vi "LabVIEW Basics #5 - Radar Sweep.vi"() -> ()   [LabVIEW 2019]
uses:
  <vilib>/picture/picture.llb/imagedata.ctl
  <vilib>/MakerHub/LINX/Public/Utilities/Open Serial.vi
  <vilib>/MakerHub/LINX/Public/Sensors/Motion/Servo/Servo Open One Channel.vi
  <vilib>/MakerHub/LINX/Public/Sensors/Motion/Servo/Servo Set Pulse Width One Channel.vi
  <vilib>/MakerHub/LINX/Public/Sensors/Motion/Servo/Servo Close One Channel.vi
  <vilib>/MakerHub/LINX/LMH-LINX.lvlib
  <vilib>/MakerHub/LINX/Public/Sensors/Motion/Servo/Servo.lvlib
  <vilib>/MakerHub/LINX/Public/Sensors/Distance/Ultrasonic/Ultrasonic.lvlib
  <vilib>/ptbypt/NI_PtbyPt.lvlib
panel:
  out "ping":bool
  out "Degrees":dbl format="%#_3f"
  out "Distance":dbl caption="CM" format="%#_2g"
  out "2D Picture":picture
  out "Device Name":string
  in  "Stop":bool
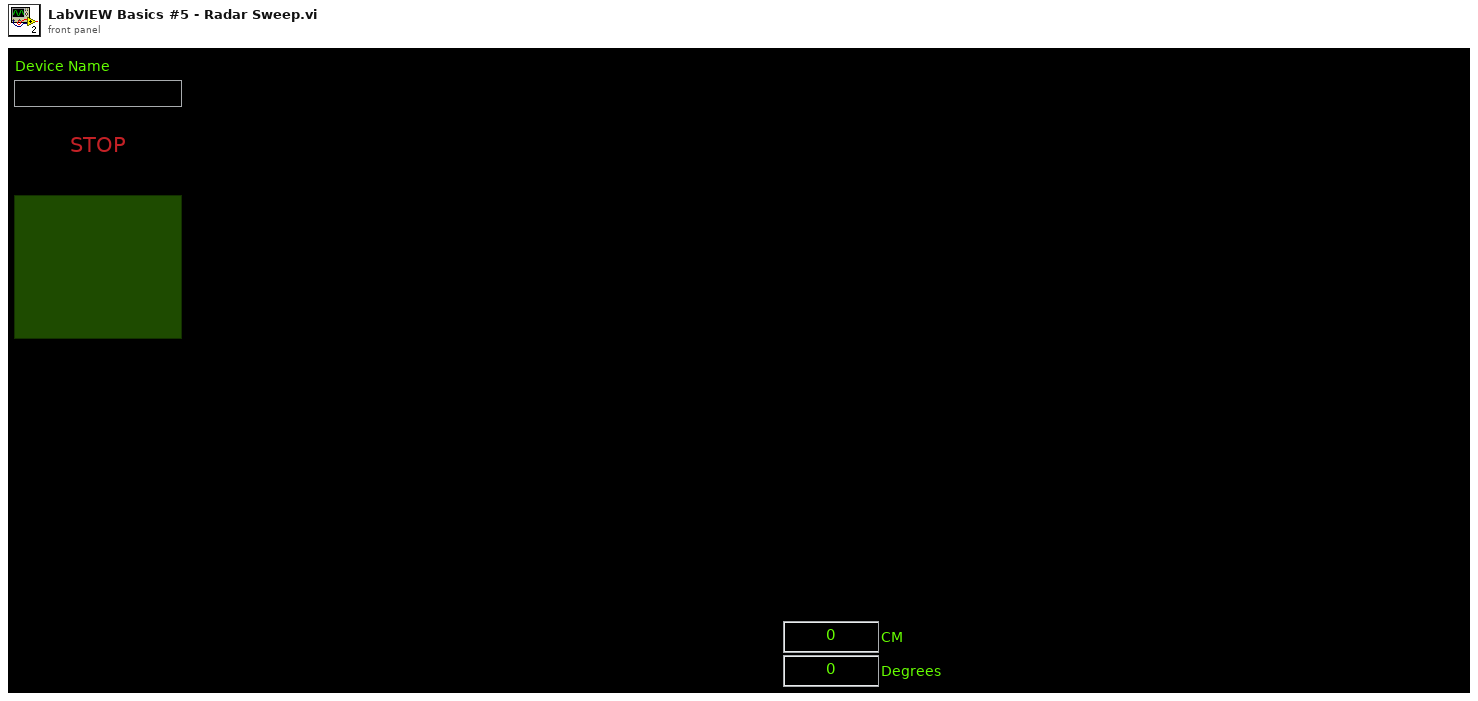
[diagram p1: front panel]
types:
  T1 = typedef "imagedata.ctl" = cluster{"image type":i32, "image depth":i32, "image":u8[], "mask":u8[], "colors":u32[], "Rectangle":cluster{"left":i16, "top":i16, "right":i16, "bottom":i16}}
  T2 = typedef "LMH-LINX.lvlib/LINX Ref.ctl" = cluster{"IO":T3, "Interface":T4, "LINX Device Config":T5}
  T3 = typedef "LMH-LINX.lvlib/Platform.ctl" = enum16{"Remote", "Local"}
  T4 = typedef "LMH-LINX.lvlib/Interface.ctl" = enum16{"Serial", "TCP"}
  T5 = typedef "LMH-LINX.lvlib/Device.lvlib/LINX Device Config.ctl" = cluster{"Interface":T4, "COM Port":refnum<visa-resource-name>, "TCP Configuration":T6, "Device Family":u8, "Device ID":u8, "Device Name":string, "TCP Ref":refnum<k5>, "Channels":T7}
  T6 = typedef "LMH-LINX.lvlib/Device.lvlib/TCP Config.ctl" = cluster{"IP Address":string, "Port":u16}
  T7 = typedef "LMH-LINX.lvlib/Channels.ctl" = cluster{"DI":u8[], "DO":u8[], "AI":u8[], "AO":u8[], "PWM":u8[], "QE":u8[], "UART":u8[], "I2C 2":u8[], "SPI":u8[], "CAN":u8[], "Servo":u8[], "AI Ref (V)":dbl, "AI Resolution (Bits)":u8, "AO Ref (V)":dbl, "AO Resolution (Bits)":u8}
  T8 = cluster{"maximum":dbl, "minimum":dbl, "clip to min":bool, "log?(F)":bool, "grid color":u32, "plot color":u32, "format and precision":cluster{"format":enum8{"Decimal", "Scientific", "Engineering", "Binary", "Octal", "Hex"}, "precision":u8}, "visible section":u16}
  T9 = typedef "LVBoundsTypeDef.ctl" = cluster{"Width":u32, "Height":u32}
  T10 = cluster{"pixel center":cluster{"x":i16, "y":i16}, "scale factors":cluster{"a":dbl, "b":dbl, "log?":bool}, "grid color":u32, "start angle":dbl, "end angle":dbl, "tick length":i16, "pixel radius":i32}
  T11 = cluster{"Distance (cm)":dbl, "Angle (Deg)":dbl}[]
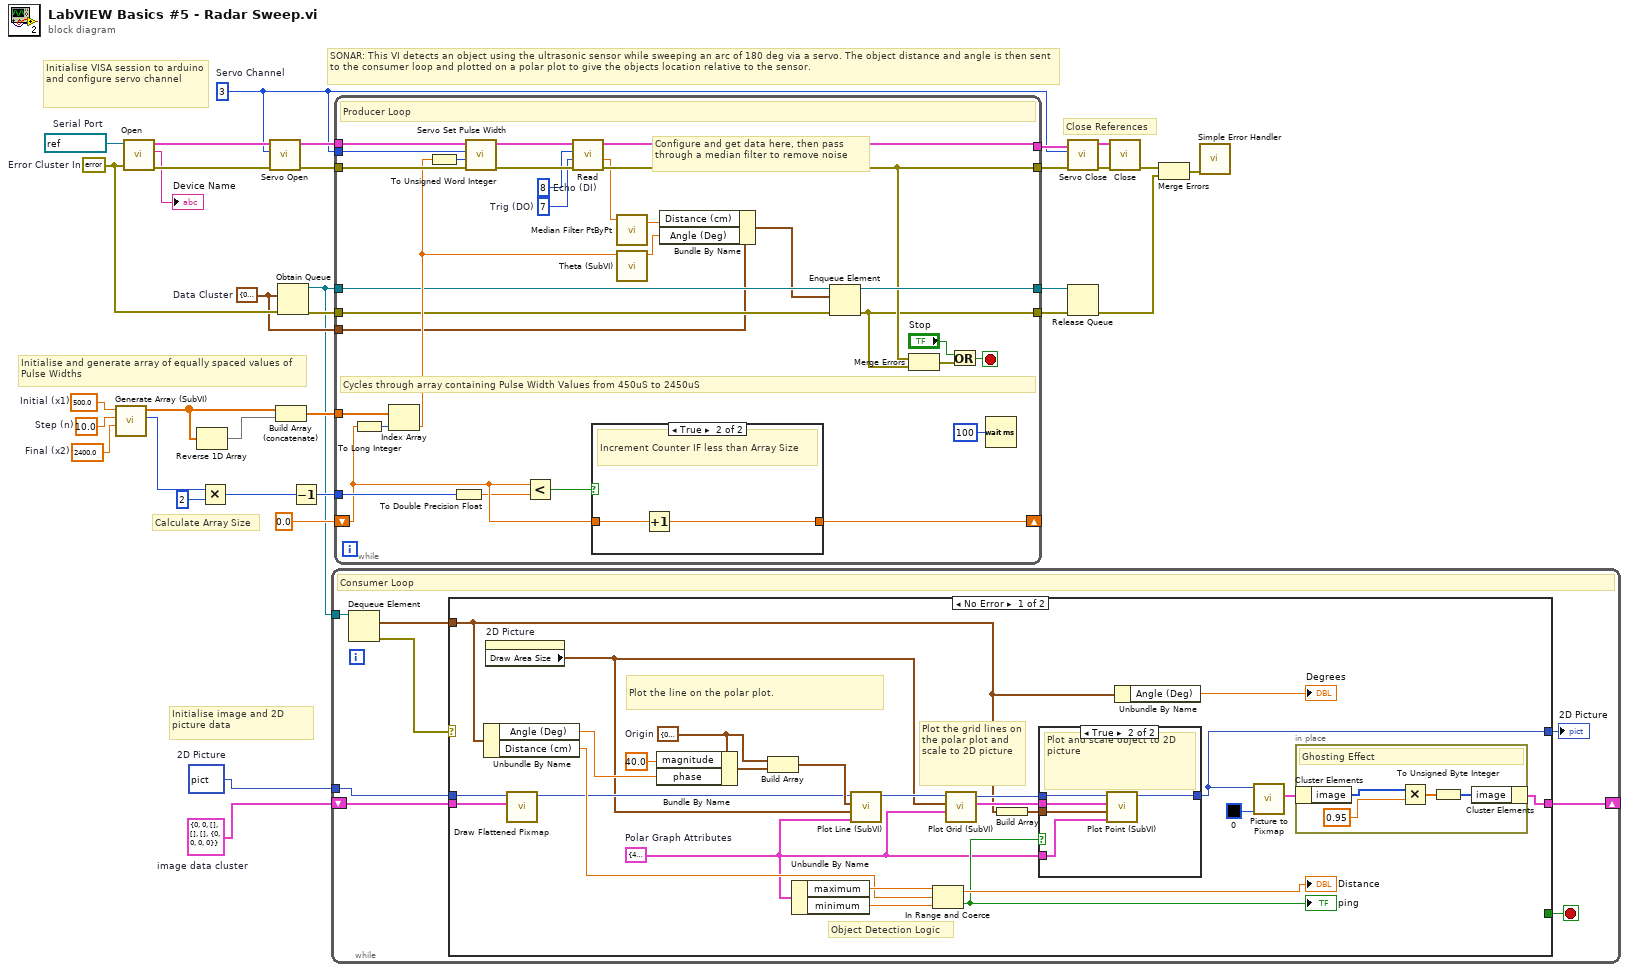
[diagram p0: block diagram]
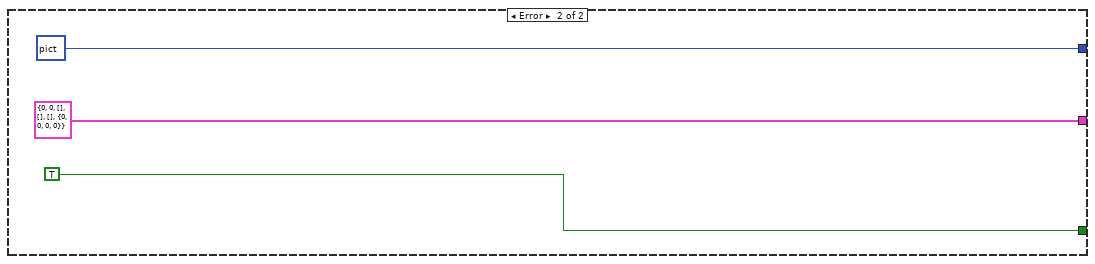
[diagram p3: hidden frame]
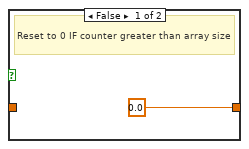
[diagram p4: hidden frame]
diagram:
  w1 = T1 {"image type"=0, "image depth"=0, "image"=[], "mask"=[], "colors"=[], "Rectangle"={"left"=0, "top"=0, "right"=0, "bottom"=0}}  # image data cluster
  w2 = picture data[5B]  # 2D Picture
  w7 = cluster{"Distance (cm)":dbl, "Angle (Deg)":dbl} {"Distance (cm)"=0.0, "Angle (Deg)"=0.0}  # Data Cluster
  w21 = 2400.0  # Final (x2)
  w20 = 10.0  # Step (n)
  w19 = 500.0  # Initial (x1)
  w24 = u8 3  # Servo Channel
  w10 = errorcluster {"status"=FALSE, "code"=0, "source"=""}  # Error Cluster In
  w33 = refnum<visa-resource-name> "COM6"  # Serial Port
  # "Initialise image and 2D picture data"
  # "Close References"
  # "Calculate Array Size"
  # "Initialise and generate array of equally spaced values of Pulse Widths"
  # "Initialise VISA session to arduino and configure servo channel"
  # "SONAR: This VI detects an object using the ultrasonic sensor while sweeping an arc of 180 deg via a servo. The object distance and angle is then sent to the consumer loop and plotted on a polar plot to give the objects location relative to the sensor."
  n1 = call "Generate Array (SubVI).vi"("Final"=w21, "Step"=w20, "Initial"=w19) -> ("Array size"=w14:i32, "Array out"=w17:dbl[])  [unwired: 6 in, 1 out]
  n2 = call-poly <vilib>:"Open.vi"("Error In"=w10, "Serial Port"=w33) -> ("Error Out"=w29:errorcluster, "Device Name"=→"Device Name":string, "LINX Resource"=w30:T2)  [unwired: 7 in]
  n3 = Reverse 1D Array(array=w17) -> (reversed array=w16:dbl[])
  n4 = Multiply(x=w14, y=2) -> (x*y=w15:i32)
  n5 = call-poly <vilib>:"Servo Open.vi"("Error In"=w29, "Servo Channel"=w24, "LINX Resource"=w30) -> ("Error Out"=w27:errorcluster, "LINX Resource"=w28:T2)  [unwired: 7 in]
  n6 = Build Array (concatenate)(w17, w16) -> (w18:dbl[])
  n7 = Obtain Queue(element data type=w7, error in (no error)=w10) -> (queue out=w3:refnum<queue>, error out=w11:errorcluster)  [unwired: 3 in, 1 out]
  n8 = Decrement(x=w15) -> (x-1=w22:i32)
  n9 = while {
    tunnel: w3 -> [w34]
    tunnel: w2 -> [w38]
    shift-right: [w35] -> _
    shift-left: w1 -> [w37]
    stop <- w39 stop-if-true
    # "Consumer Loop"
    n10 = Dequeue Element(queue=w34) -> (element=w40:cluster{"Distance (cm)":dbl, "Angle (Deg)":dbl}, error out=w41:errorcluster)  [unwired: 2 in, 2 out]
    n11 = case shown="No Error" w41 {
      tunnel: w40 -> [w49 _]
      tunnel: [_ TRUE] -> w39
      tunnel: w38 -> [w66 _]
      tunnel: w37 -> [w65 _]
      tunnel: [w61 picture data[5B] ("new picture")] -> w36
      tunnel: [w64 T1 {"image type"=0, "image depth"=0, "image"=[], "mask"=[], "colors"=[], "Rectangle"={"left"=0, "top"=0, "right"=0, "bottom"=0}} ("image data")] -> w35
      frame No Error {
        w47 = T8 {"maximum"=40.0, "minimum"=2.0, "clip to min"=TRUE, "log?(F)"=FALSE, "grid color"=9868950, "plot color"=65280, "format and precision"={"format"=enum."Decimal", "precision"=0}, "visible section"=4}  # Polar Graph Attributes
        w43 = cluster{"magnitude":dbl, "phase":dbl} {"magnitude"=0.0, "phase"=0.0}  # Origin
        # "Object Detection Logic"
        # "Plot the line on the polar plot."
        # "Plot the grid lines on the polar plot and scale to 2D picture"
        n12 = Unbundle By Name(w49) -> ("Angle (Deg)"=w54:dbl, "Distance (cm)"=w55:dbl)
        n13 = property on="2D Picture" class="Pict"() -> ("Draw Area Size"=w51:T9)  [unwired: 2 in, 2 out]
        n14 = call <vilib>:"Draw Flattened Pixmap.vi"("image data"=w65, "picture"=w66) -> ("new picture"=w52:picture)  [unwired: 7 in]
        n15 = Bundle By Name(cluster=w43, "magnitude"=40.0, "phase"=w54) -> (w42:cluster{"magnitude":dbl, "phase":dbl})
        n16 = Build Array(w43, w42) -> (w62:cluster{"magnitude":dbl, "phase":dbl}[])
        n17 = Unbundle By Name(w47) -> ("maximum"=w57:dbl, "minimum"=w56:dbl)
        n18 = call "Plot Line (SubVI).vi"("Polar Graph Attributes"=w47, "Draw Area Size"=w51, "Polar Array"=w62, "new picture in"=w52) -> ("new picture out"=w63:picture)  [unwired: 7 in]
        n19 = In Range and Coerce(upper limit=w57, x=w55, lower limit=w56) -> (coerced(x)=→"Distance":dbl, In Range?=w53:bool)
        "ping" <- w53
        n20 = call "Plot Grid (SubVI).vi"("Polar Graph Attributes"=w47, "Draw Area Size"=w51, "new picture in"=w63) -> ("grid measurements"=w59:T10, "new picture out"=w60:picture)  [unwired: 7 in]
        n21 = Build Array(w49) -> (w50:T11)
        n22 = case shown="True" w53 {
          tunnel: w50 -> [_ w72]
          tunnel: [w71 w76] -> w61
          tunnel: w60 -> [w71 w74]
          tunnel: w59 -> [_ w73]
          tunnel: w47 -> [_ w75]
          frame False {
            # "Nothing Detected"
          }
          frame True {
            # "Plot and scale object to 2D picture"
            n23 = call "Plot Point (SubVI).vi"("Polar Graph Attributes"=w75, "Array"=w72, "grid measurements"=w73, "new picture in"=w74) -> ("new picture"=w76:picture)  [unwired: 7 in]
          }
        }
        n24 = Unbundle By Name(w49) -> ("Angle (Deg)"=→"Degrees":dbl)
        n25 = call <vilib>:"Picture to Pixmap.vi"("Background Color"=u32 0, "picture"=w61) -> ("image data"=w46:T1)  [unwired: 8 in, 1 out]
        n26 = in-place {
          # "Ghosting Effect"
          n27 = in-place-cluster #1(w46) -> ("image"=w70:u8[])
          n28 = Multiply(x=w70, y=0.95) -> (x*y=w68:dbl[])
          n29 = To Unsigned Byte Integer(number=w68) -> (unsigned 8bit integer=w67:u8[])
          n30 = in-place-cluster #1("image"=w67) -> (w64:T1)
        }
      }
      frame Error {
      }
    }
    "2D Picture" <- w36
  }
  n31 = while {
    tunnel: [w101] -> w32
    tunnel: [w88] -> w31
    tunnel: w28 -> [w103]
    tunnel: w27 -> [w104]
    tunnel: w24 -> [w109]
    tunnel: w18 -> [w108]
    shift-right: [w97] -> _
    shift-left: 0.0 -> [w106]
    tunnel: w22 -> [w107]
    tunnel: w7 -> [w91]
    tunnel: w11 -> [w95]
    tunnel: [w87] -> w8
    tunnel: w3 -> [w94]
    tunnel: [w93] -> w9
    stop <- w110 stop-if-true
    w98 = u8 7  # Trig (DO)
    w99 = u8 8  # Echo (DI)
    # "Configure and get data here, then pass through a median filter to remove noise"
    # "Cycles through array containing Pulse Width Values from 450uS to 2450uS"
    # "Producer Loop"
    n32 = To Long Integer(number=w106) -> (32bit integer=w83:i32)
    n33 = Index Array "Index Array"(array=w108, index=w83) -> (element=w96:dbl)
    n34 = To Unsigned Word Integer(number=w96) -> (unsigned 16bit integer=w84:u16)
    n35 = To Double Precision Float(number=w107) -> (double precision float=w82:dbl)
    n36 = call-poly <vilib>:"Servo Set Pulse Width.vi"("Error In"=w104, "Pulse Width (uS)"=w84, "Servo Channel"=w109, "LINX Resource"=w103) -> ("Error Out"=w100:errorcluster, "LINX Resource"=w102:T2)  [unwired: 6 in]
    n37 = Less?(x=w106, y=w82) -> (x < y?=w105:bool)
    n38 = call <vilib>:"Read.vi"("Error In"=w100, "DO Channel"=w98, "DI Channel"=w99, "LINX Resource"=w102) -> ("Error Out"=w88:errorcluster, "Centimeters"=w80:dbl, "LINX Resource"=w101:T2)  [unwired: 4 in, 1 out]
    n39 = case shown="True" w105 {
      tunnel: [0.0 w113] -> w97
      tunnel: w106 -> [_ w112]
      frame False {
        # "Reset to 0 IF counter greater than array size"
      }
      frame True {
        # "Increment Counter IF less than Array Size"
        n40 = Increment(x=w112) -> (x+1=w113:dbl)
      }
    }
    n41 = call <vilib>:"Median Filter PtByPt.vi"("x"=w80) -> ("Filtered x"=w81:dbl)  [unwired: 3 in, 1 out]
    n42 = call "Theta (SubVI).vi"("PWM"=w96) -> ("Theta"=w92:dbl)  [unwired: 9 in, 1 out]
    n43 = Bundle By Name(cluster=w91, "Distance (cm)"=w81, "Angle (Deg)"=w92) -> (w90:cluster{"Distance (cm)":dbl, "Angle (Deg)":dbl})
    n44 = Enqueue Element(queue=w94, element=w90, error in (no error)=w95) -> (queue out=w93:refnum<queue>, error out=w87:errorcluster)  [unwired: 1 in, 1 out]
    n45 = Merge Errors(w88, w87) -> (w86:errorcluster)
    n46 = Or(x="Stop", y=w86) -> (x .or. y?=w110:bool)
    n47 = Wait (ms)(milliseconds to wait=u32 100 ("Slide")) -> ()  [unwired: 1 out]
  }
  n48 = call-poly <vilib>:"Servo Close.vi"("Error In"=w31, "Servo Channel"=w24, "LINX Resource"=w32) -> ("Error Out"=w26:errorcluster, "LINX Resource"=w25:T2)  [unwired: 7 in]
  n49 = Release Queue(queue=w9, error in (no error)=w8) -> (error out=w4:errorcluster)  [unwired: 1 in, 2 out]
  n50 = call <vilib>:"Close.vi"("Error In"=w26, "LINX Resource"=w25) -> ("Error Out"=w6:errorcluster)  [unwired: 9 in]
  n51 = Merge Errors(w6, w4) -> (w5:errorcluster)
  n52 = call <vilib>:"Simple Error Handler.vi"("error in (no error)"=w5) -> ()  [unwired: 4 in, 5 out]
